vi "phy_packet_gen.vi"(11 "Input bytes":u8[](array[numeric])) -> (3 "output bit stream":i8[](array[numeric]))   [LabVIEW 2014]
uses:
  <vilib>/addons/Modulation/Digital/Support/Controls/Pack Bits Parameters.ctl
  <vilib>/addons/Modulation/niDMT.lvlib
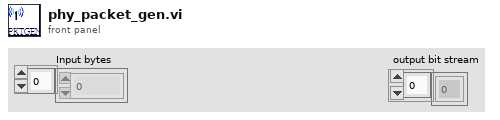
[diagram p1: front panel]
types:
  T1 = typedef "niDMT.lvlib/Pack Bits Parameters.ctl" = enum16{"Unsigned", "Signed"}
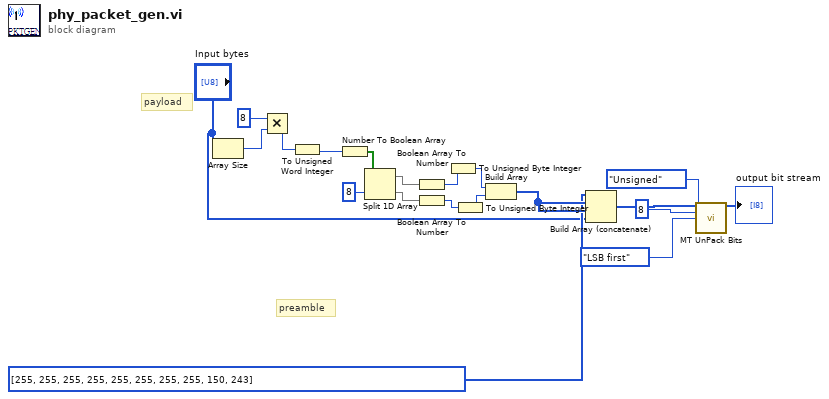
[diagram p0: block diagram]
diagram:
  # "payload"
  # "preamble"
  n1 = Array Size(array="Input bytes") -> (size(s)=w20:i32)
  n2 = Multiply(x=8, y=w20) -> (x*y=w18:i32)
  n3 = To Unsigned Word Integer(number=w18) -> (unsigned 16bit integer=w17:u16)
  n4 = Number To Boolean Array(number=w17) -> (Boolean array=w16:bool[])
  n5 = Split 1D Array(array=w16, index=8) -> (first subarray=w15:bool[], second subarray=w14:bool[])
  n6 = Boolean Array To Number(Boolean array=w15) -> (number=w11:u32)
  n7 = Boolean Array To Number(Boolean array=w14) -> (number=w10:u32)
  n8 = To Unsigned Byte Integer(number=w11) -> (unsigned 8bit integer=w8:u8)
  n9 = To Unsigned Byte Integer(number=w10) -> (unsigned 8bit integer=w9:u8)
  n10 = Build Array(w8, w9) -> (w13:u8[])
  n11 = Build Array (concatenate)(u8[] [255, 255, 255, 255, 255, 255, 255, 255, 150, 243], w13, w13, "Input bytes") -> (w6:u8[])
  n12 = call <vilib>:"MT UnPack Bits.vi"("input integers"=w6, "bits per integer"=8, "packed bit order"=enum16{"MSB first", "LSB first"}."LSB first", "integer format"=Pack_Bits_Parameters."Unsigned") -> ("output bit stream"=→"output bit stream":i8[])  [unwired: 10 in, 1 out]
